vi "Get Encoder.vi"(8 "error in (no error)":errorcluster, 11 "Motor in":refnum<class "Motor.lvclass">) -> (0 "error out":errorcluster, 2 "encoder pos in display unit":dbl, 3 "Motor out":refnum<class "Motor.lvclass">)   [LabVIEW 2016, in "Hardware.lvlib" / "Motor.lvlib" / "Motor.lvclass"]
uses:
  <userlib>/Common Components/Hardware/Motor/Motor/Motor.lvclass
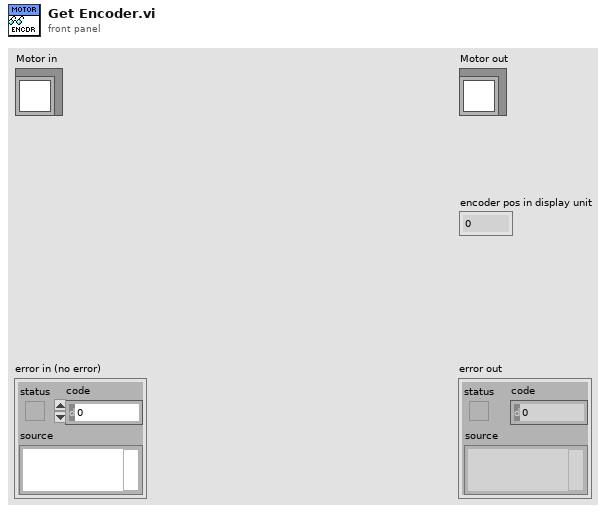
[diagram p1: front panel]
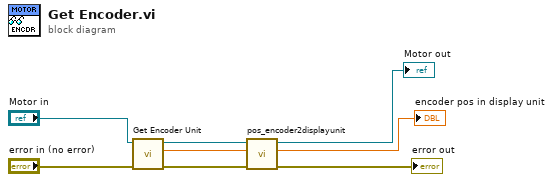
[diagram p0: block diagram]
diagram:
  n1 = call-dynamic "Get Encoder Unit.vi"("error in (no error)"="error in (no error)", "Motor in"="Motor in") -> ("error out"=w7:errorcluster, "encoder (unit)"=w2:dbl, "Motor out"=w4:refnum<class "Motor.lvclass">)  [unwired: 7 in]
  n2 = call <userlib>:"pos_encoder2displayunit.vi"("error in (no error)"=w7, "encoder (unit)"=w2, "Motor in"=w4) -> ("error out"=→"error out":errorcluster, "pos in display unit"=→"encoder pos in display unit":dbl, "Motor out"=→"Motor out":refnum<class "Motor.lvclass">)  [unwired: 6 in]
